vi "水温校准.vi"() -> ()   [LabVIEW 2016, in "斯坦道多参数.lvlib"]
uses:
  <vilib>/Utility/config.llb/NI_LVConfig.lvlib
panel:
  in  "补偿后温度值":dbl
  out "电极温度读值":dbl
  in  "温度偏移补偿":dbl
  in  "温度电极选择":enum16{"pH电极", "电导率电极", "溶解氧电极", "浊度电极"}(ring)
  # "温度电极设定"
  # "℃"
  # "℃"
  # "℃"
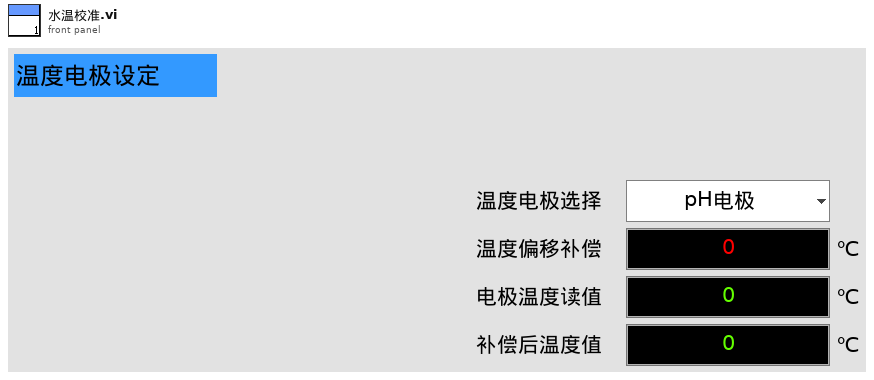
[diagram p1: front panel]
types:
  T1 = typedef "NI_LVConfig.lvlib/Config Data RefNum.ctl" = refnum<k1>
  T2 = cluster{"pH探头选择":u16, "DO探头选择":u16, "电导率探头选择":u16, "浊度探头选择":u16, "叶绿素a探头选择":u16, "蓝绿藻探头选择":u16}
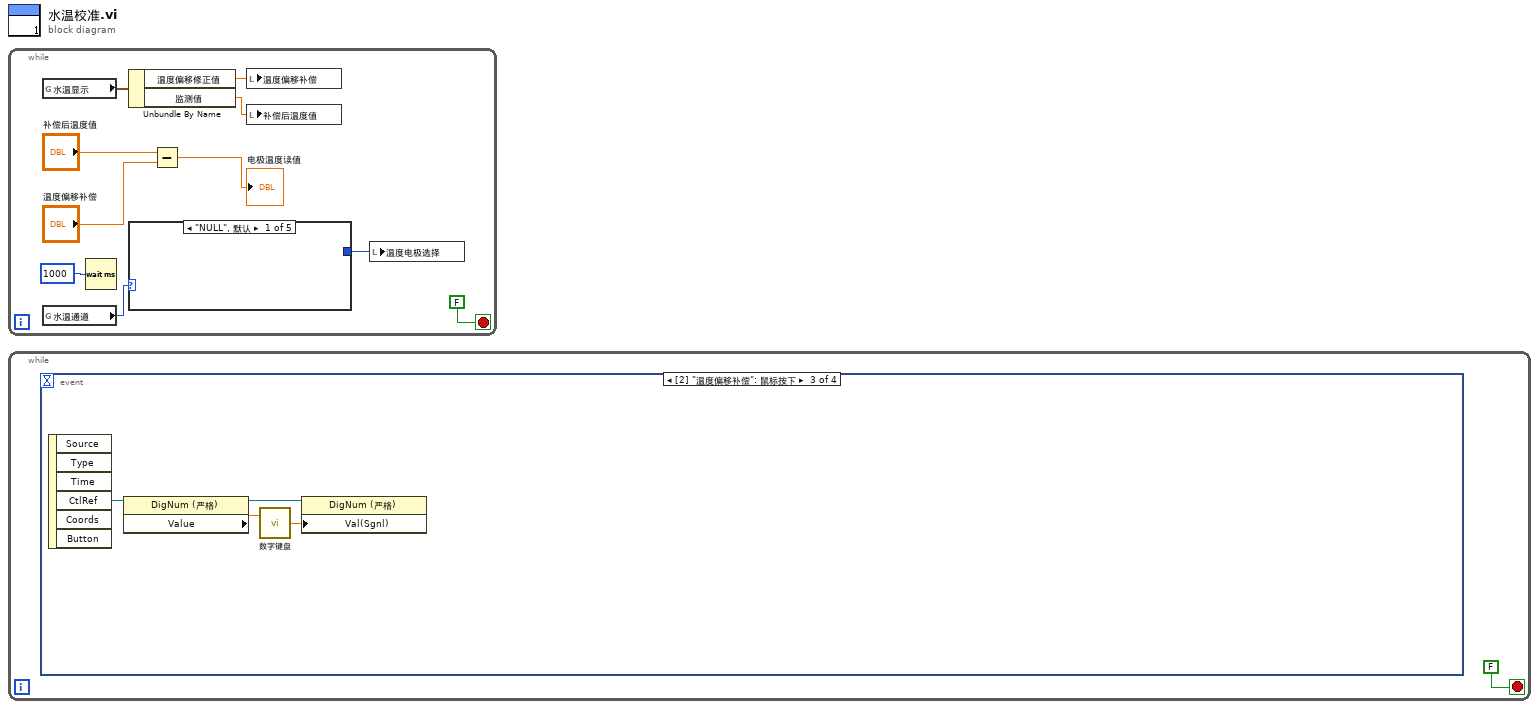
[diagram p0: block diagram]
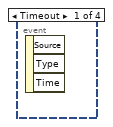
[diagram p2: hidden frame]
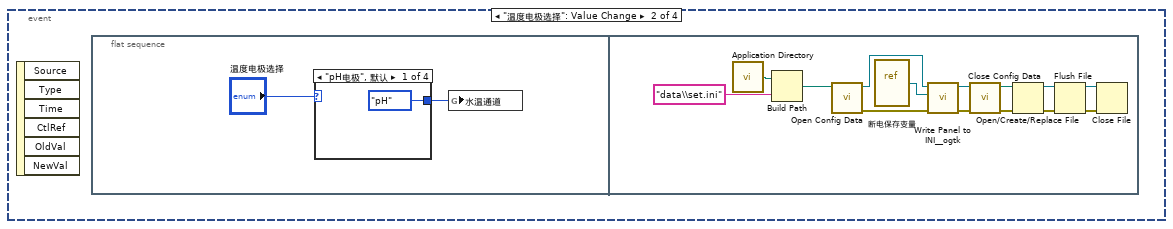
[diagram p3: hidden frame]
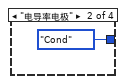
[diagram p4: hidden frame]
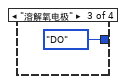
[diagram p5: hidden frame]
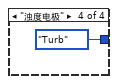
[diagram p6: hidden frame]
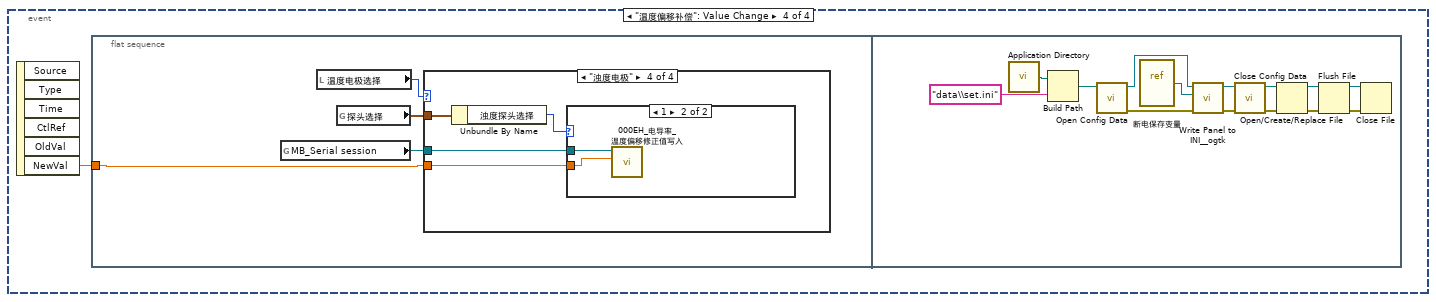
[diagram p7: hidden frame]
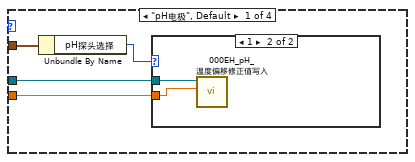
[diagram p8: hidden frame]
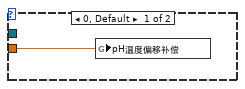
[diagram p9: hidden frame]
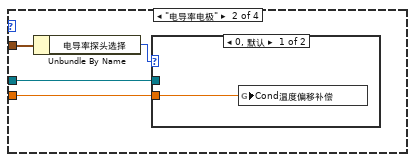
[diagram p10: hidden frame]
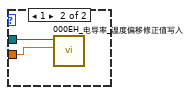
[diagram p11: hidden frame]
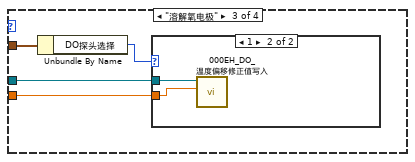
[diagram p12: hidden frame]
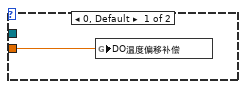
[diagram p13: hidden frame]
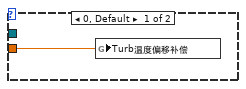
[diagram p14: hidden frame]
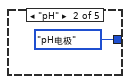
[diagram p15: hidden frame]
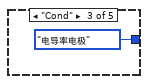
[diagram p16: hidden frame]
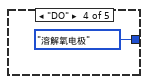
[diagram p17: hidden frame]
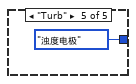
[diagram p18: hidden frame]
diagram:
  n1 = while {
    stop <- FALSE stop-if-true
    n2 = global read "多参数全局变量.vi" "水温显示"() -> (w1:cluster{"CH":u16, "监测值":dbl, "温度偏移修正值":sgl})
    n3 = global read "断电保存变量.vi" "水温通道"() -> (w3:enum16{"NULL", "pH", "Cond", "DO", "Turb"})
    n4 = Wait (ms)(milliseconds to wait=u32 1000 ("等待时间（毫秒）")) -> ()  [unwired: 1 out]
    n5 = Unbundle By Name(w1) -> ("温度偏移修正值"=w5:sgl, "监测值"=w4:dbl)
    n6 = case shown="\"NULL\", 默认" w3 {
      tunnel: [_ enum16{"pH电极", "电导率电极", "溶解氧电极", "浊度电极"}."pH电极" ("温度电极选择") enum16{"pH电极", "电导率电极", "溶解氧电极", "浊度电极"}."电导率电极" ("温度电极选择") enum16{"pH电极", "电导率电极", "溶解氧电极", "浊度电极"}."溶解氧电极" ("温度电极选择") enum16{"pH电极", "电导率电极", "溶解氧电极", "浊度电极"}."浊度电极" ("温度电极选择")] -> w2
      frame "NULL", Default {
      }
      frame "pH" {
      }
      frame "Cond" {
      }
      frame "DO" {
      }
      frame "Turb" {
      }
    }
    n7 = Subtract(x="补偿后温度值", y="温度偏移补偿") -> (x-y=→"电极温度读值":dbl)
    n8 = local write "温度偏移补偿"(w5) -> ()
    n9 = local write "补偿后温度值"(w4) -> ()
    n10 = local write "温度电极选择"(w2) -> ()
  }
  n11 = while {
    stop <- FALSE stop-if-true
    n12 = event shown="[2] \"温度偏移补偿\": 鼠标按下" {
      selector: _ -> [_ _ _ _]
      dyn-events: _ -> [_ _ _ _]
      timeout: _ -> [_ _ _ _]
      event Timeout {
        n13 = event-data() -> ()  [unwired: 1 in, 3 out]
      }
      event "温度电极选择": Value Change {
        n14 = event-data() -> ()  [unwired: 1 in, 6 out]
        n15 = flat-sequence {
          frame #0 {
            n16 = case shown="\"pH电极\", 默认" "温度电极选择" {
              tunnel: [enum16{"NULL", "pH", "Cond", "DO", "Turb"}."pH" ("水温通道") enum16{"NULL", "pH", "Cond", "DO", "Turb"}."Cond" ("水温通道") enum16{"NULL", "pH", "Cond", "DO", "Turb"}."DO" ("水温通道") enum16{"NULL", "pH", "Cond", "DO", "Turb"}."Turb" ("水温通道")] -> w17
              frame "pH电极", Default {
              }
              frame "电导率电极" {
              }
              frame "溶解氧电极" {
              }
              frame "浊度电极" {
              }
            }
            n17 = global write "断电保存变量.vi" "水温通道"(w17) -> ()
          }
          frame #1 {
            n18 = call <vilib>:"Application Directory.vi"() -> ("Application Directory"=w31:path)
            n19 = Build Path(base path=w31, name or relative path="data\\set.ini" ("名称或相对路径")) -> (appended path=w30:path)
            n20 = call <vilib>:"Open Config Data.vi"("configuration file path"=w30) -> ("error out"=w34:errorcluster, "refnum"=w35:T1)  [unwired: 8 in, 1 out]
            n21 = vi-ref "断电保存变量.vi"() -> (w28:refnum<vi>)
            n22 = call <userlib>:"Write Panel to INI__ogtk.vi"("error in (no error)"=w34, "VI ref"=w28, "refnum"=w35) -> ("error out"=w32:errorcluster, "refnum out"=w33:T1)  [unwired: 7 in]
            n23 = call <vilib>:"Close Config Data.vi"("error in (no error)"=w32, "refnum"=w33) -> ("error out"=w24:errorcluster, "file path"=w25:path)  [unwired: 8 in]
            n24 = Open/Create/Replace File(file path (use dialog)=w25, error in=w24) -> (refnum out=w26:refnum<file>, error out=w27:errorcluster)  [unwired: 4 in, 1 out]
            n25 = Flush File(refnum=w26, error in=w27) -> (refnum out=w22:refnum<file>, error out=w23:errorcluster)
            n26 = Close File(refnum=w22, error in=w23) -> ()  [unwired: 2 out]
          }
        }
      }
      event "温度偏移补偿": Mouse Down {
        n27 = event-data() -> ("CtlRef"=w39:refnum<vi>)  [unwired: 1 in, 5 out]
        n28 = property class="DigNum (严格)"(reference=w39) -> (reference out=w36:refnum<vi>, "Value"=w38:dbl)  [unwired: 1 in, 1 out]
        n29 = call "数字键盘.vi"("OldNumber"=w38) -> ("NewNumber"=w37:dbl)  [unwired: 1 in]
        n30 = property class="DigNum (严格)"(reference=w36, "Val(Sgnl)"=w37) -> ()  [unwired: 1 in, 2 out]
      }
      event "温度偏移补偿": Value Change {
        n31 = event-data() -> ("NewVal"=w40:dbl)  [unwired: 1 in, 5 out]
        n32 = flat-sequence {
          tunnel: w40 -> [w43]
          frame #0 {
            n33 = global read "多参数全局变量.vi" "MB_Serial session"() -> (w42:refnum<class "MB_Master_Serial.lvclass">)
            n34 = local read "温度电极选择"() -> (w44:enum16{"pH电极", "电导率电极", "溶解氧电极", "浊度电极"})
            n35 = global read "断电保存变量.vi" "探头选择"() -> (w41:T2)
            n36 = case shown="\"浊度电极\"" w44 {
              tunnel: w43 -> [w48 w55 w62 w69]
              tunnel: w42 -> [w47 w54 w59 w66]
              tunnel: w41 -> [w46 w53 w61 w68]
              frame "pH电极", Default {
                n37 = Unbundle By Name(w46) -> ("pH探头选择"=w45:u16)
                n38 = case shown="1" w45 {
                  tunnel: w48 -> [w49 w51]
                  tunnel: w47 -> [_ w50]
                  frame 0, Default {
                    n39 = global write "断电保存变量.vi" "pH温度偏移补偿"(w49) -> ()
                  }
                  frame 1 {
                    n40 = call "000EH_pH_温度偏移修正值写入.vi"("数值"=w51, "MB_Serial session in"=w50) -> ()  [unwired: 8 in, 2 out]
                  }
                }
              }
              frame "电导率电极" {
                n41 = Unbundle By Name(w53) -> ("电导率探头选择"=w52:u16)
                n42 = case shown="0, 默认" w52 {
                  tunnel: w55 -> [w56 w58]
                  tunnel: w54 -> [_ w57]
                  frame 0, Default {
                    n43 = global write "断电保存变量.vi" "Cond温度偏移补偿"(w56) -> ()
                  }
                  frame 1 {
                    n44 = call "000EH_电导率_温度偏移修正值写入.vi"("数值"=w58, "MB_Serial session in"=w57) -> ()  [unwired: 8 in, 2 out]
                  }
                }
              }
              frame "溶解氧电极" {
                n45 = Unbundle By Name(w61) -> ("DO探头选择"=w60:u16)
                n46 = case shown="1" w60 {
                  tunnel: w62 -> [w63 w64]
                  tunnel: w59 -> [_ w65]
                  frame 0, Default {
                    n47 = global write "断电保存变量.vi" "DO温度偏移补偿"(w63) -> ()
                  }
                  frame 1 {
                    n48 = call "000EH_DO_温度偏移修正值写入.vi"("数值"=w64, "MB_Serial session in"=w65) -> ()  [unwired: 8 in, 2 out]
                  }
                }
              }
              frame "浊度电极" {
                n49 = Unbundle By Name(w68) -> ("浊度探头选择"=w67:u16)
                n50 = case shown="1" w67 {
                  tunnel: w69 -> [w70 w72]
                  tunnel: w66 -> [_ w71]
                  frame 0, Default {
                    n51 = global write "断电保存变量.vi" "Turb温度偏移补偿"(w70) -> ()
                  }
                  frame 1 {
                    n52 = call "000EH_电导率_温度偏移修正值写入.vi"("数值"=w72, "MB_Serial session in"=w71) -> ()  [unwired: 8 in, 2 out]
                  }
                }
              }
            }
          }
          frame #1 {
            n53 = call <vilib>:"Application Directory.vi"() -> ("Application Directory"=w82:path)
            n54 = Build Path(base path=w82, name or relative path="data\\set.ini" ("名称或相对路径")) -> (appended path=w81:path)
            n55 = call <vilib>:"Open Config Data.vi"("configuration file path"=w81) -> ("error out"=w85:errorcluster, "refnum"=w86:T1)  [unwired: 8 in, 1 out]
            n56 = vi-ref "断电保存变量.vi"() -> (w79:refnum<vi>)
            n57 = call <userlib>:"Write Panel to INI__ogtk.vi"("error in (no error)"=w85, "VI ref"=w79, "refnum"=w86) -> ("error out"=w83:errorcluster, "refnum out"=w84:T1)  [unwired: 7 in]
            n58 = call <vilib>:"Close Config Data.vi"("error in (no error)"=w83, "refnum"=w84) -> ("error out"=w75:errorcluster, "file path"=w76:path)  [unwired: 8 in]
            n59 = Open/Create/Replace File(file path (use dialog)=w76, error in=w75) -> (refnum out=w77:refnum<file>, error out=w78:errorcluster)  [unwired: 4 in, 1 out]
            n60 = Flush File(refnum=w77, error in=w78) -> (refnum out=w73:refnum<file>, error out=w74:errorcluster)
            n61 = Close File(refnum=w73, error in=w74) -> ()  [unwired: 2 out]
          }
        }
      }
    }
  }
